vi "network_scan.vi"() -> ()   [LabVIEW 2015]
panel:
  out "Array 2":errorcluster[](array[cluster])
  out "Array":string[](array[string])
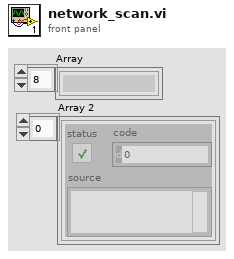
[diagram p1: front panel]
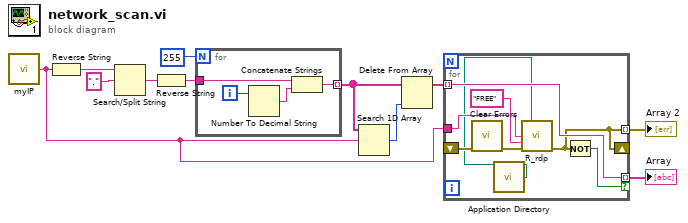
[diagram p0: block diagram]
diagram:
  n1 = call "myIP.vi"() -> ("My IP"=w1:string)  [unwired: 1 in]
  n2 = Reverse String(1:w1) -> (0:w10:string)
  n3 = Search/Split String(string=w10, search string/char (-)=".") -> (match + rest of string=w8:string)  [unwired: 1 in, 2 out]
  n4 = Reverse String(1:w8) -> (0:w7:string)
  n5 = for {
    N: 255 -> [_]
    tunnel: w7 -> [w14]
    tunnel: [w12] -> w5 mode=indexing
    i -> [w15]
    n6 = Number To Decimal String(number=w15) -> (decimal integer string=w13:string)  [unwired: 1 in]
    n7 = Concatenate Strings(w14, w13) -> (w12:string)
  }
  n8 = Search 1D Array(1D array=w5, element=w1) -> (index of element=w6:i32)  [unwired: 1 in]
  n9 = Delete From Array(array=w5, index=w6) -> (array with subset deleted=w4:string[])  [unwired: 1 in, 1 out]
  n10 = for {
    tunnel: w4 -> [w20] mode=indexing
    shift-right: [w18] -> _
    shift-left: _ -> [w22]
    tunnel: [w18] -> w2 mode=indexing
    tunnel: [w20] -> w3 mode=indexing if=w19
    tunnel: w1 -> [w17]
    n11 = call <vilib>:"Clear Errors.vi"("error in (no error)"=w22) -> ("error out"=w21:errorcluster)  [unwired: 5 in, 1 out]
    n12 = call <vilib>:"Application Directory.vi"() -> ("Application Directory"=w16:path)
    n13 = call "R_rdp.vi"("install path"=w16, "Ip"=w17, "Name in"="FREE", "error in (no error)"=w21) -> ("error out"=w18:errorcluster)  [unwired: 9 in, 2 out]
    n14 = Not(x=w18) -> (.not. x?=w19:bool)
  }
  "Array" <- w3
  "Array 2" <- w2
